vi "Poll.FG.vi"(7 "Action":T4, 8 "error in":errorcluster, 10 "Selected Channels":T1, 11 "Parent Ref":T5=18446744073709551615 format="%.0x") -> (0 "error out":errorcluster, 2 "Selected Channels out":T1, 3 "Parent Ref Out":T5=18446744073709551615 format="%.0x")   [LabVIEW 2019, in "Diagnostics Addon System Explorer.lvlib"]
uses:
  Diagnostics Addon System Explorer.lvlib
  <vilib>/NI VeriStand/Custom Device API/Custom Device Item Ref.ctl
  Types/Poll.Settings.ctl
  Types/Poll.LinkedNode.ctl
  Addon Shared/Types/DPID.Rate.ctl
  Types/FG.Action.ctl
  Addon Shared/SubVIs/Constants.vi
  <vilib>/NI VeriStand/Custom Device API/Set Item Property (Dependent Node Pointer).vi
  <vilib>/NI VeriStand/Custom Device API/Set Item Property (String Array).vi
  <vilib>/NI/NI VeriStand Advanced SysDef API/_SubVIs/SysDef.Property.Set.U32.vi
  <vilib>/NI VeriStand/Custom Device API/Get Item Property (String Array).vi
  <vilib>/NI VeriStand/Custom Device API/Get Item Property (Dependent Node Pointer).vi
  <vilib>/NI VeriStand/Custom Device API/Get Item Property (U32).vi
  <vilib>/NI VeriStand/Custom Device API/Custom Device API.lvlib
  Addon Shared/Diagnostics Addon Shared.lvlib
  <vilib>/NI/NI VeriStand Advanced SysDef API/SysDef API/Advanced System Definition.lvlib
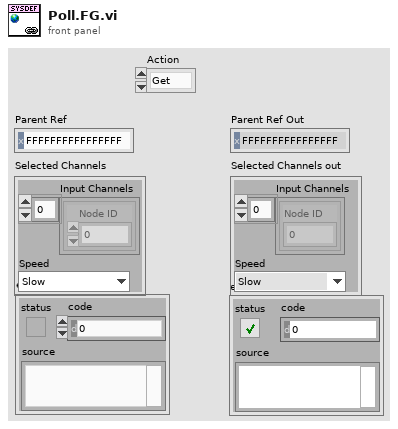
[diagram p1: front panel]
types:
  T1 = typedef "Diagnostics Addon System Explorer.lvlib/Poll.Settings.ctl" = cluster{"Input Channels":T2[], "Speed":T3}
  T2 = typedef "Diagnostics Addon System Explorer.lvlib/Poll.LinkedNode.ctl" = cluster{"Node ID":u64}
  T3 = typedef "Diagnostics Addon Shared.lvlib/DPID.Rate.ctl" = enum16{"Slow", "Medium", "Fast"}
  T4 = typedef "Diagnostics Addon System Explorer.lvlib/FG.Action.ctl" = enum16{"Get", "Set"}
  T5 = typedef "Custom Device API.lvlib/Custom Device Item Ref.ctl" = u64
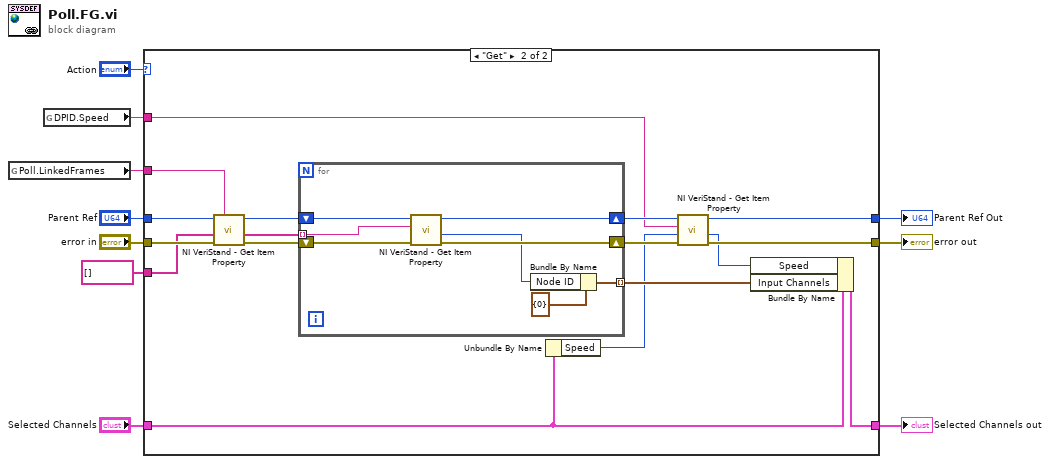
[diagram p0: block diagram]
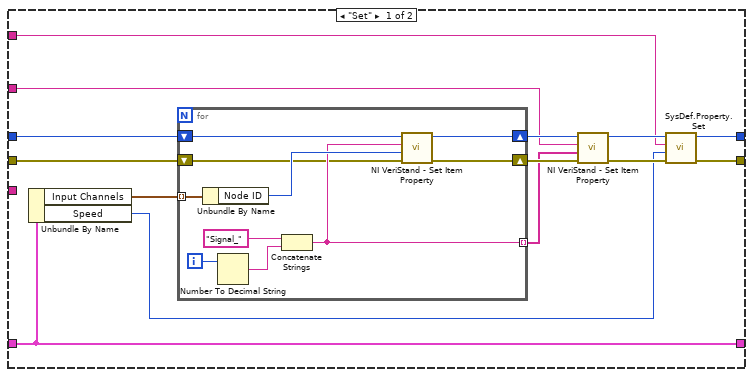
[diagram p2: hidden frame]
diagram:
  n1 = global read "Constants.vi" "Poll.LinkedFrames"() -> (w2:string)
  n2 = global read "Constants.vi" "DPID.Speed"() -> (w1:string)
  n3 = case shown="\"Get\"" "Action" {
    tunnel: "error in" -> [w20 w51]
    tunnel: "Parent Ref" -> [w19 w50]
    tunnel: w2 -> [w18 w49]
    tunnel: string[] [] -> [_ w48]
    tunnel: "Selected Channels" -> [w17 w38]
    tunnel: [w17 w45] -> w7
    tunnel: [w16 w41] -> w6
    tunnel: [w13 w39] -> w5
    tunnel: w1 -> [w12 w36]
    frame "Set" {
      n4 = Unbundle By Name(w17) -> ("Input Channels"=w24:T2[], "Speed"=w11:T3)
      n5 = for {
        tunnel: w24 -> [w31] mode=indexing
        tunnel: [w29] -> w21 mode=indexing
        shift-right: [w27] -> w23
        shift-left: w20 -> [w28]
        shift-right: [w25] -> w22
        shift-left: w19 -> [w26]
        i -> [w33]
        n6 = Unbundle By Name(w31) -> ("Node ID"=w30:u64)
        n7 = Number To Decimal String(number=w33) -> (decimal integer string=w32:string)  [unwired: 1 in]
        n8 = Concatenate Strings("Signal_" ("string"), w32) -> (w29:string)
        n9 = call-poly <vilib>:"NI VeriStand - Set Item Property.vi"("error in (no error)"=w28, "Dependent Node Ref"=w30, "Property Name"=w29, "Item Ref in"=w26) -> ("error out"=w27:errorcluster, "Item Ref out"=w25:T5)  [unwired: 5 in, 1 out]
      }
      n10 = call-poly <vilib>:"NI VeriStand - Set Item Property.vi"("error in (no error)"=w23, "Value"=w21, "Property Name"=w18, "Item Ref in"=w22) -> ("error out"=w15:errorcluster, "Item Ref out"=w14:T5)  [unwired: 5 in, 1 out]
      n11 = call-poly <vilib>:"SysDef.Property.Set.vi"("error in (no error)"=w15, "Value"=w11, "Property Name"=w12, "nodeID"=w14) -> ("error out"=w16:errorcluster, "nodeID out"=w13:u64)  [unwired: 6 in]
    }
    frame "Get" {
      n12 = call-poly <vilib>:"NI VeriStand - Get Item Property.vi"("error in (no error)"=w51, "Default Value"=w48, "Property Name"=w49, "Item Ref in"=w50) -> ("error out"=w47:errorcluster, "Value"=w44:string[], "Item Ref out"=w46:T5)  [unwired: 4 in, 1 out]
      n13 = for {
        shift-right: [w57] -> w40
        shift-left: w46 -> [w58]
        tunnel: w44 -> [w56] mode=indexing
        shift-right: [w55] -> w42
        shift-left: w47 -> [w59]
        tunnel: [w53] -> w43 mode=indexing
        n14 = call-poly <vilib>:"NI VeriStand - Get Item Property.vi"("error in (no error)"=w59, "Property Name"=w56, "Item Ref in"=w58) -> ("error out"=w55:errorcluster, "Dependent Node Ref"=w54:T5, "Item Ref out"=w57:T5)  [unwired: 5 in, 1 out]
        n15 = Bundle By Name(cluster=T2 {"Node ID"=0} ("MonitoredChannelSettings"), "Node ID"=w54) -> (w53:T2)
      }
      n16 = Unbundle By Name(w38) -> ("Speed"=w37:T3)
      n17 = call-poly <vilib>:"NI VeriStand - Get Item Property.vi"("error in (no error)"=w42, "Default Value"=w37, "Property Name"=w36, "Item Ref in"=w40) -> ("error out"=w41:errorcluster, "Value"=w35:u32, "Item Ref out"=w39:T5)  [unwired: 4 in, 1 out]
      n18 = Bundle By Name(cluster=w38, "Speed"=w35, "Input Channels"=w43) -> (w45:T1)
    }
  }
  "error out" <- w6
  "Parent Ref Out" <- w5
  "Selected Channels out" <- w7
